vi "Detect_Particle-9.vi"(4 "[IN] Image Filtering Settings":T1, 5 "Keep Nega-\ntive Values?":bool, 6 "# Channel":u8, 7 "Particle Searching Settings":T4 {"Type of particle filter"."Measurement Parameter" items=["Center of Mass X", "Center of Mass Y", "First Pixel X", "First Pixel Y", "Bounding Rect Left", "Bounding Rect Top", "Bounding Rect Right", "Bounding Rect Bottom", "Max Feret Diameter Start X", "Max Feret Diameter Start Y", "Max Feret Diameter End X", "Max Feret Diameter End Y", "Max Horiz. Segment Length Left", "Max Horiz. Segment Length Right", "Max Horiz. Segment Length Row", "-", "Bounding Rect Width", "Bounding Rect Height", "Bounding Rect Diagonal", "Perimeter", "Convex Hull Perimeter", "Holes' Perimeter", "Max Feret Diameter", "Equivalent Ellipse Major Axis", "Equivalent Ellipse Minor Axis", "Equivalent Ellipse Minor Axis (Feret)", "Equivalent Rect Long Side", "Equivalent Rect Short Side", "Equivalent Rect Diagonal", "Equivalent Rect Short Side (Feret)", "Average Horiz. Segment Length", "Average Vert. Segment Length", "Hydraulic Radius", "Waddel Disk Diameter", "-", "Area", "Holes' Area", "Particle & Holes' Area", "Convex Hull Area", "Image Area", "-", "Number of Holes", "Number of Horiz. Segments", "Number of Vert. Segments", "-", "Orientation", "Max Feret Diameter Orientation", "-", "% Area/Image Area", "% Area/(Particle & Holes' Area)", "Ratio of Equivalent Ellipse Axes", "Ratio of Equivalent Rect Sides", "-", "Elongation Factor", "Compactness Factor", "Heywood Circularity Factor", "Type Factor", "-", "Sum X", "Sum Y", "Sum XX", "Sum XY", "Sum YY", "Sum XXX", "Sum XXY", "Sum XYY", "Sum YYY", "-", "Moment of Inertia XX", "Moment of Inertia XY", "Moment of Inertia YY", "Moment of Inertia XXX", "Moment of Inertia XXY", "Moment of Inertia XYY", "Moment of Inertia YYY", "Norm. Moment of Inertia XX", "Norm. Moment of Inertia XY", "Norm. Moment of Inertia YY", "Norm. Moment of Inertia XXX", "Norm. Moment of Inertia XXY", "Norm. Moment of Inertia XYY", "Norm. Moment of Inertia YYY", "Hu Moment 1", "Hu Moment 2", "Hu Moment 3", "Hu Moment 4", "Hu Moment 5", "Hu Moment 6", "Hu Moment 7"]}, 8 "error IN":errorcluster, 9 "[IN] Binarization Settings":cluster{"MinBin2":sgl, "MaxBin2":sgl}[](array[cluster]), 10 "[IN] Destination Image":T2, 11 "[IN] Frame":T2) -> (0 "error OUT":errorcluster, 2 "[OUT] Particle Reports (Pixels)":T5(array[cluster]) {"Orientation" format="%.2f"; "Dimensions"."Height" format="%.2f"; "Dimensions"."Width" format="%.2f"; "Center of Mass"."Y" format="%.2f"; "Center of Mass"."X" format="%.2f"; "Bounding Rect"."Bottom" format="%.2f"; "Bounding Rect"."Right" format="%.2f"; "Bounding Rect"."Top" format="%.2f"; "Bounding Rect"."Left" format="%.2f"; "Number of Holes" format="%.2f"; "Area" format="%.2f"}, 3 "[OUT] Binarized Image":T2)   [LabVIEW 2013]
doc: "SubVI demonstrates the resulting localization of particles with selected parameters\nPerfoming: \n- binarization\n- particle filters (Feret diameters)\nOutput: \n- Particle report (center of mass) + Area"
uses:
  <vilib>/vision/Image Controls.llb/IMAQ Image.ctl
  <vilib>/vision/NI_Vision_Development_Module.lvlib
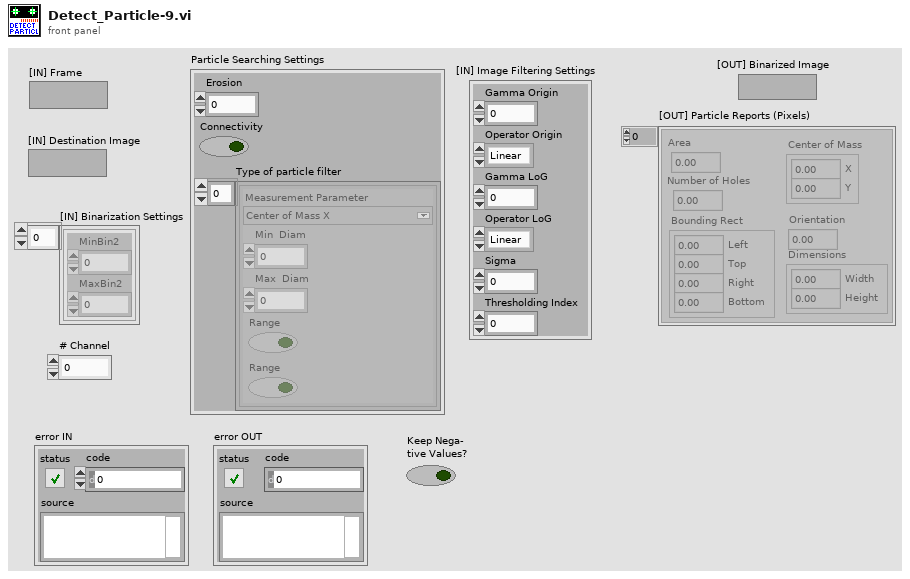
[diagram p1: front panel]
types:
  T1 = cluster{"Gamma Origin":sgl, "Operator Origin":enum32{"Linear", "Log", "Exp", "Square", "Square root", "Power X", "Power 1/X"}, "Gamma LoG":sgl, "Operator LoG":enum32{"Linear", "Log", "Exp", "Square", "Square root", "Power X", "Power 1/X"}, "Sigma":dbl, "Thresholding Index":i8}
  T2 = typedef "IMAQ Image.ctl" = refnum<image>
  T3 = typedef "Particle Parameters" = i32
  T4 = cluster{"Erosion":i32, "Connectivity ":bool, "Type of particle filter":cluster{"Measurement Parameter":T3, "Min  Diam":dbl, "Max  Diam":dbl, "Range":bool, "Range":bool}[]}
  T5 = cluster{"Area":dbl, "Number of Holes":dbl, "Bounding Rect":cluster{"Left":dbl, "Top":dbl, "Right":dbl, "Bottom":dbl}, "Center of Mass":cluster{"X":dbl, "Y":dbl}, "Orientation":dbl, "Dimensions":cluster{"Width":dbl, "Height":dbl}}[]
  T6 = cluster{"Starting Value":sgl, "Incremental Value":sgl, "Histogram":u32[]}
  T7 = cluster{"Measurement Parameter":T3, "Min  Diam":dbl, "Max  Diam":dbl, "Range":bool, "Range":bool}[]
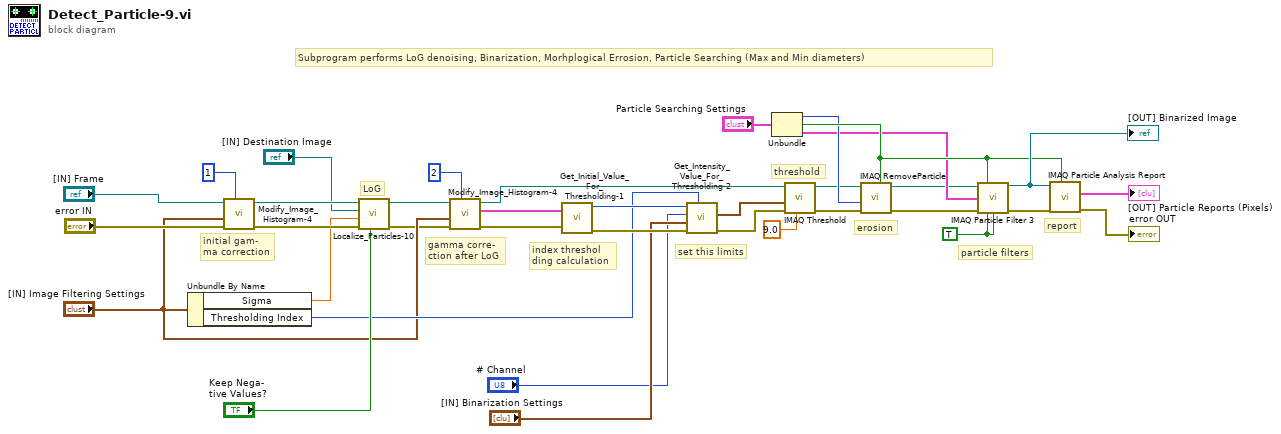
[diagram p0: block diagram]
diagram:
  w36 = TRUE ("Fill Holes? (F)")
  # "report"
  # "erosion"
  # "particle filters"
  # "threshold"
  # "set this limits"
  # "index threshol\nding calculation"
  # "gamma corre-\nction after LoG"
  # "LoG"
  # "initial gam-\nma correction"
  # "Subprogram performs LoG denoising, Binarization, Morhplogical Errosion, Particle Searching (Max and Min diameters)"
  n1 = Unbundle By Name("[IN] Image Filtering Settings") -> ("Sigma"=w16:dbl, "Thresholding Index"=w10:i8)
  n2 = call "Modify_Image_Histogram-4.vi"("1 - Origin\n2 - LoG"=u8 1 ("1 - Origin\n2 - LoG"), "error IN"="error IN", "[IN] Image Filtering Settings"="[IN] Image Filtering Settings", "[IN] LoG Processed Image"="[IN] Frame") -> ("error OUT"=w21:errorcluster, "[OUT] Histogram Modified Image"=w18:T2)  [unwired: 5 in, 1 out]
  n3 = call "Localize_Particles-10.vi"("Keep Nega-\ntive Values?"="Keep Nega-\ntive Values?", "error IN"=w21, "[IN] Sigma"=w16, "[IN] Destination Image"="[IN] Destination Image", "[IN] Frame"=w18) -> ("error OUT"=w1:errorcluster, "[OUT] LoG Processed Image"=w14:T2)  [unwired: 3 in, 1 out]
  n4 = call "Modify_Image_Histogram-4.vi"("1 - Origin\n2 - LoG"=u8 2 ("1 - Origin\n2 - LoG"), "error IN"=w1, "[IN] Image Filtering Settings"="[IN] Image Filtering Settings", "[IN] LoG Processed Image"=w14) -> ("error OUT"=w4:errorcluster, "[OUT] Histogram"=w5:T6, "[OUT] Histogram Modified Image"=w6:T2)  [unwired: 5 in]
  n5 = call "Get_Initial_Value_For_Thresholding-1.vi"("[IN] Histogram Graph"=w5, "error IN"=w4) -> ("[OUT] Index of starting \npoint for thresholding"=w13:i32, "error OUT"=w12:errorcluster)  [unwired: 2 out]
  n6 = call "Get_Intensity_Value_For_Thresholding-2.vi"("[IN] Index for \nthresholding"=w10, "error IN"=w12, "[IN] Binarization Set\ntings (Both Channels)"="[IN] Binarization Settings", "[IN] 1 or 2 channel"="# Channel", "[IN] Index of starting \npoint for thresholding"=w13) -> ("error OUT"=w7:errorcluster, "[OUT] For Operator \nBinarization Values"=w8:cluster{"MinBin2":sgl, "MaxBin2":sgl})  [unwired: 1 in, 1 out]
  n7 = Unbundle("Particle Searching Settings") -> ("Erosion"=w30:i32, "Connectivity"=w31:bool, "Type of particle filter"=w29:T7)
  n8 = call "IMAQ Threshold"("Replace Value"=sgl 9.0, "error in (no error)"=w7, "Range"=w8, "Image Src"=w6) -> ("error out"=w26:errorcluster, "Image Dst Out"=w25:T2)  [unwired: 6 in]
  n9 = call "IMAQ RemoveParticle"("Connectivity 4/8 (8)"=w31, "error in (no error)"=w26, "Number of Erosion"=w30, "Image Src"=w25) -> ("error out"=w27:errorcluster, "Image Dst Out"=w28:T2)  [unwired: 6 in]
  n10 = call "IMAQ Particle Filter 3"("Image Src"=w28, "Connectivity 4/8 (8)"=w31, "Selection Values"=w29, "error in (no error)"=w27, "Reject Border? (F)"=w36, "Fill Holes? (F)"=w36) -> ("Image Dst Out"=w35:T2, "error out"=w34:errorcluster)  [unwired: 7 in, 1 out]
  "[OUT] Binarized Image" <- w35
  n11 = call "IMAQ Particle Analysis Report"("Connectivity 4/8 (8)"=w31, "error in (no error)"=w34, "Image"=w35) -> ("error out"=→"error OUT":errorcluster, "Particle Reports (Pixels)"=→"[OUT] Particle Reports (Pixels)":T5)  [unwired: 3 in, 4 out]
